vi "Register Values.vi"(8 "error in (no error)":errorcluster, 9 "Calib/Offset Register (0:OFSTA)":u32(ring) items=["OFSTA", "OFSTB", "OG", "OB", "SR", "SX", "TYG", "TYB", "MYG", "MYB", "TZR", "TZX", "MZR", "MZX", "TSTDR", "TSTDX", "MSTDR", "MSTDX"], 10 "Registers (0:A)":u32(ring) items=["A", "B", "C", "D", "E", "F", "G", "H", "I", "J", "RA", "RB", "RC", "RD", "RE", "RF", "RG", "RH", "RI", "RJ", "RK", "RL"], 11 "VISA resource name":refnum<visa-resource-name>) -> (0 "error out":errorcluster, 1 "Offset/Calib Register Data":dbl[](array[numeric]) format="%.2f", 2 "Register Data":dbl[](array[numeric]) format="%^.3e", 3 "VISA resource name out":refnum<visa-resource-name>, 4 "Offset Valid Array Items":i32, 5 "Valid Array Items":i32)   [LabVIEW 2017, in "Agilent 4194.lvlib"]
doc: "This function outputs the instrument's array register data."
uses:
  Agilent 4194.lvlib
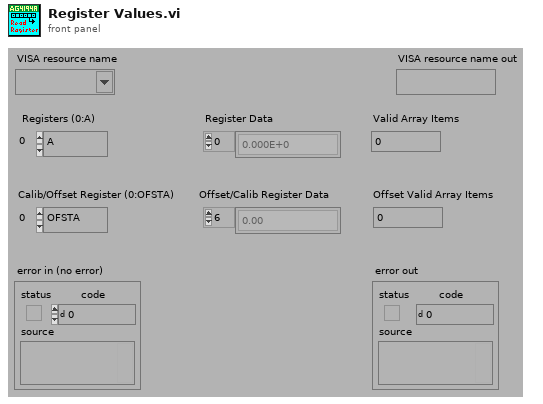
[diagram p1: front panel]
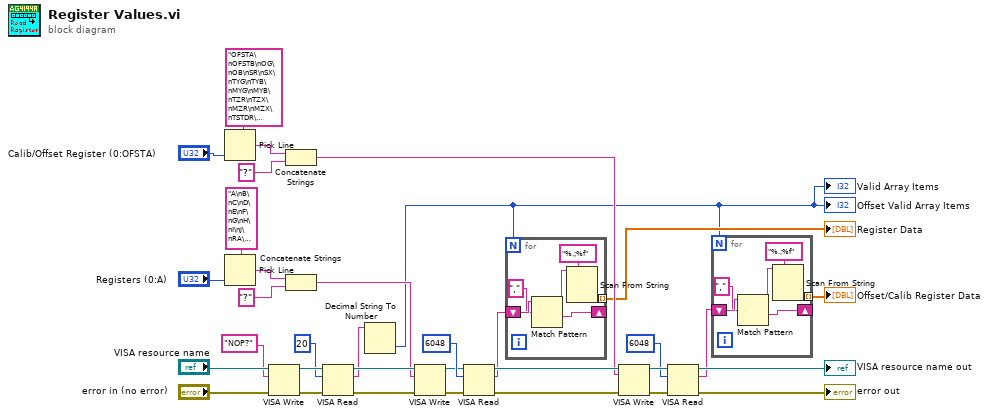
[diagram p0: block diagram]
diagram:
  n1 = Pick Line(multi-line string="OFSTA\nOFSTB\nOG\nOB\nSR\nSX\nTYG\nTYB\nMYG\nMYB\nTZR\nTZX\nMZR\nMZX\nTSTDR\nTSTDX\nMSTDR\nMSTDX", line index="Calib/Offset Register (0:OFSTA)") -> (output string=w12:string)  [unwired: 1 in]
  n2 = Pick Line(multi-line string="A\nB\nC\nD\nE\nF\nG\nH\nI\nJ\nRA\nRB\nRC\nRD\nRE\nRF\nRG\nRH\nRI\nRJ\nRK\nRL", line index="Registers (0:A)") -> (output string=w22:string)  [unwired: 1 in]
  n3 = VISA Write(VISA resource name="VISA resource name", write buffer="NOP?" ("write buffer (\"\")"), error in (no error)="error in (no error)") -> (VISA resource name out=w33:refnum<visa-resource-name>, error out=w34:errorcluster)  [unwired: 1 out]
  n4 = Concatenate Strings(w12, "?" ("output string")) -> (w10:string)
  n5 = Concatenate Strings(w22, "?" ("output string")) -> (w19:string)
  n6 = VISA Read(VISA resource name=w33, byte count=u32 20 ("byte count (0)"), error in (no error)=w34) -> (VISA resource name out=w28:refnum<visa-resource-name>, read buffer=w1:string, error out=w27:errorcluster)  [unwired: 1 out]
  n7 = Decimal String To Number(string=w1) -> (number=w2:i32)  [unwired: 2 in, 1 out]
  "Offset Valid Array Items" <- w2
  "Valid Array Items" <- w2
  n8 = VISA Write(VISA resource name=w28, write buffer=w19, error in (no error)=w27) -> (VISA resource name out=w30:refnum<visa-resource-name>, error out=w29:errorcluster)  [unwired: 1 out]
  n9 = VISA Read(VISA resource name=w30, byte count=u32 6048 ("byte count (0)"), error in (no error)=w29) -> (VISA resource name out=w15:refnum<visa-resource-name>, read buffer=w8:string, error out=w14:errorcluster)  [unwired: 1 out]
  n10 = for {
    N: w2 -> [_]
    shift-right: [w35] -> _
    shift-left: w8 -> [w39]
    tunnel: [w36] -> w7 mode=indexing
    n11 = Match Pattern(string=w39, regular expression="," ("search char (-)")) -> (before substring=w37:string, after substring=w35:string)  [unwired: 1 in, 2 out]
    n12 = Scan From String(format string="%.;%f", input string=w37) -> (output 1=w36:dbl)  [unwired: 3 in, 3 out]
  }
  "Register Data" <- w7
  n13 = VISA Write(VISA resource name=w15, write buffer=w10, error in (no error)=w14) -> (VISA resource name out=w17:refnum<visa-resource-name>, error out=w18:errorcluster)  [unwired: 1 out]
  n14 = VISA Read(VISA resource name=w17, byte count=u32 6048 ("byte count (0)"), error in (no error)=w18) -> (VISA resource name out=→"VISA resource name out":refnum<visa-resource-name>, read buffer=w4:string, error out=→"error out":errorcluster)  [unwired: 1 out]
  n15 = for {
    N: w2 -> [_]
    shift-right: [w41] -> _
    shift-left: w4 -> [w45]
    tunnel: [w42] -> w3 mode=indexing
    n16 = Match Pattern(string=w45, regular expression="," ("search char (-)")) -> (before substring=w43:string, after substring=w41:string)  [unwired: 1 in, 2 out]
    n17 = Scan From String(format string="%.;%f", input string=w43) -> (output 1=w42:dbl)  [unwired: 3 in, 3 out]
  }
  "Offset/Calib Register Data" <- w3
